vi "getBeamName.vi"(10 "Holo:":dbl) -> (1 "just beam name":string, 3 "beam name and index":string)   [LabVIEW 2022 SP3]
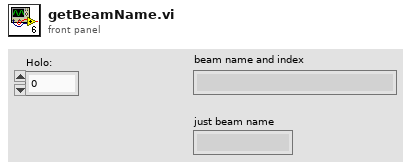
[diagram p1: front panel]
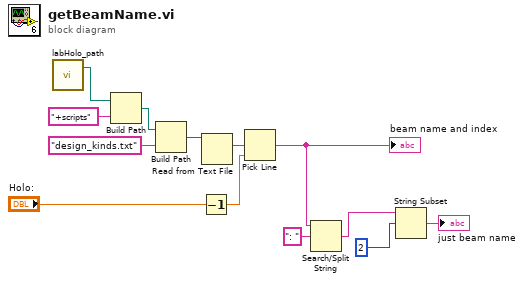
[diagram p0: block diagram]
diagram:
  n1 = call "labHolo_path.vi"() -> ("labHolo path"=w6:path)  [unwired: 2 in, 1 out]
  n2 = Build Path(base path=w6, name or relative path="+scripts") -> (appended path=w7:path)
  n3 = Build Path(base path=w7, name or relative path="design_kinds.txt") -> (appended path=w13:path)
  n4 = Decrement(x="Holo:") -> (x-1=w11:dbl)
  n5 = Read from Text File(file (use dialog)=w13) -> (text=w10:string)  [unwired: 3 in, 3 out]
  n6 = Pick Line(multi-line string=w10, line index=w11) -> (output string=w3:string)  [unwired: 1 in]
  "beam name and index" <- w3
  n7 = Search/Split String(string=w3, search string/char (-)=": ") -> (match + rest of string=w2:string)  [unwired: 1 in, 2 out]
  n8 = String Subset(string=w2, offset (0)=2) -> (substring=→"just beam name":string)  [unwired: 1 in]
